vi "Send email.vi"(8 "error in (no error)":errorcluster, 9 "message":string, 10 "attachments":path[](array[path]), 11 "email settings":T1={"email service"="smtp.gmail.com:587", "maint. email"="ivanildo@lna.br", "admin email"="frodrigues@lna.br", "S4ICS email"="s4ics@lna.br", "S4ICS login"="s4ics@lna.br", "S4ICS password"="se4RFVgy&8", "email enabled"=TRUE}) -> (0 "error out":errorcluster, 1 "fail":bool)   [LabVIEW 2018]
uses:
  <vilib>/smtpClient/Set Message Text.vi
  <vilib>/smtpClient/LabVIEWSMTPClient.lvlib
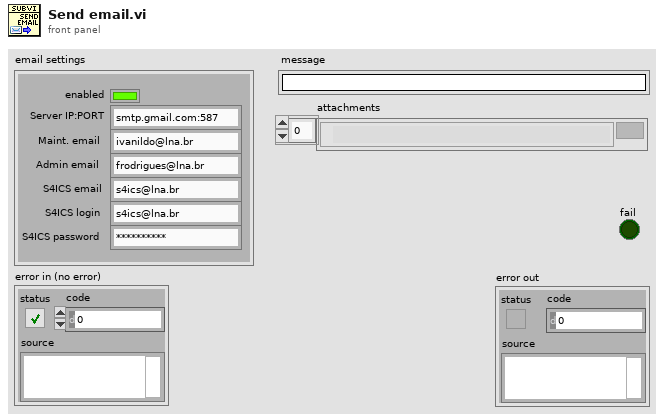
[diagram p1: front panel]
types:
  T1 = cluster{"email service":string, "maint. email":string, "admin email":string, "S4ICS email":string, "S4ICS login":string, "S4ICS password":string, "email enabled":bool}
  T2 = typedef "LabVIEWSMTPClient.lvlib/SmtpClientHandle.ctl" = refnum<k1>
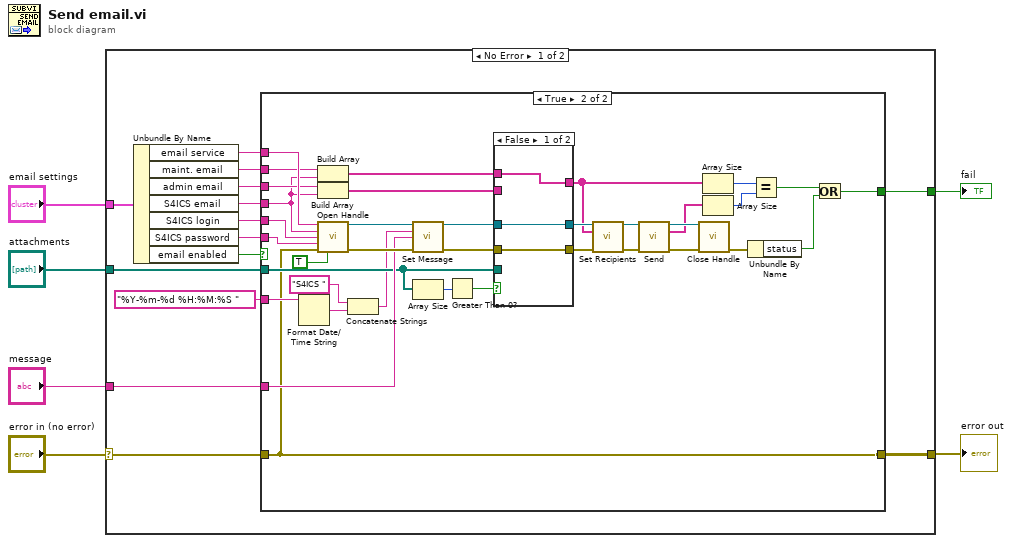
[diagram p0: block diagram]
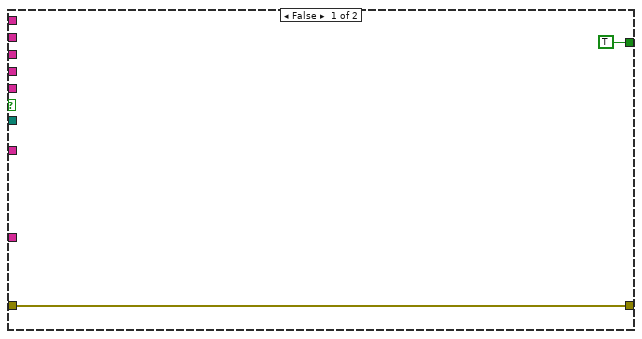
[diagram p2: hidden frame]
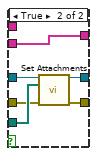
[diagram p3: hidden frame]
diagram:
  n1 = case shown="No Error" "error in (no error)" {
    selector: "error in (no error)" -> [w18 w67]
    tunnel: [w19 w67] -> w5
    tunnel: [w20 _] -> w4
    tunnel: "email settings" -> [w17 _]
    tunnel: "message" -> [w11 _]
    tunnel: "attachments" -> [w10 _]
    frame No Error {
      n2 = Unbundle By Name(w17) -> ("email service"=w15:string, "maint. email"=w9:string, "admin email"=w8:string, "S4ICS email"=w14:string, "S4ICS login"=w13:string, "S4ICS password"=w12:string, "email enabled"=w16:bool)
      n3 = case shown="True" w16 {
        tunnel: [TRUE w52] -> w20
        tunnel: [w22 w27] -> w19
        tunnel: w18 -> [w22 w27]
        tunnel: w15 -> [_ w47]
        tunnel: w14 -> [_ w37]
        tunnel: w13 -> [_ w49]
        tunnel: w12 -> [_ w48]
        tunnel: w11 -> [_ w46]
        tunnel: w10 -> [_ w44]
        tunnel: w9 -> [_ w38]
        tunnel: w8 -> [_ w39]
        tunnel: "%Y-%m-%d %H:%M:%S " ("time format string (%c)") -> [_ w29]
        frame False {
        }
        frame True {
          n4 = Format Date/Time String(time format string (%c)=w29) -> (date/time string=w31:string)  [unwired: 2 in]
          n5 = Build Array(w38, w37) -> (w35:string[])
          n6 = Build Array(w39, w37) -> (w36:string[])
          n7 = call <vilib>:"Open Handle.vi"("server address"=w47, "from"=w37, "username"=w49, "password"=w48, "error in (no error)"=w27, "use TLS (false)"=TRUE) -> ("handle out"=w33:T2, "error out"=w56:errorcluster)  [unwired: 8 in]
          n8 = Concatenate Strings("S4ICS " ("assunto:"), w31) -> (w28:string)
          n9 = call-poly <vilib>:"Set Message.vi"("handle in"=w33, "subject"=w28, "plain text message"=w46) -> ("handle out"=w32:T2)  [unwired: 11 in, 1 out]
          n10 = Array Size(array=w44) -> (size(s)=w45:i32)
          n11 = Greater Than 0?(x=w45) -> (x > 0?=w43:bool)
          n12 = case shown="False" w43 {
            tunnel: w56 -> [w59 w65]
            tunnel: w32 -> [w60 w64]
            tunnel: w44 -> [_ w66]
            tunnel: [w59 w63] -> w25
            tunnel: [w60 w62] -> w41
            tunnel: w36 -> [_ w61]
            tunnel: w35 -> [w58 _]
            tunnel: [w58 w61] -> w34
            frame False {
            }
            frame True {
              n13 = call <vilib>:"Set Attachments.vi"("handle in"=w64, "attachments"=w66, "error in (no error)"=w65) -> ("handle out"=w62:T2, "error out"=w63:errorcluster)  [unwired: 11 in]
            }
          }
          n14 = call <vilib>:"Set Recipients.vi"("handle in"=w41, "to"=w34, "error in (no error)"=w25) -> ("handle out"=w40:T2, "error out"=w42:errorcluster)  [unwired: 11 in]
          n15 = call <vilib>:"Send.vi"("handle in"=w40, "error in (no error)"=w42) -> ("handle out"=w57:T2, "invalid recipients"=w26:string[], "error out"=w24:errorcluster)  [unwired: 11 in]
          n16 = call <vilib>:"Close Handle.vi"("handle in"=w57, "error in (no error)"=w24) -> ("error out"=w51:errorcluster)  [unwired: 12 in, 1 out]
          n17 = Array Size(array=w34) -> (size(s)=w55:i32)
          n18 = Array Size(array=w26) -> (size(s)=w54:i32)
          n19 = Unbundle By Name(w51) -> ("status"=w50:bool)
          n20 = Equal?(x=w55, y=w54) -> (x = y?=w53:bool)
          n21 = Or(x=w53, y=w50) -> (x .or. y?=w52:bool)
        }
      }
    }
    frame Error {
    }
  }
  "fail" <- w4
  "error out" <- w5
